vi "SetRange_XDM3051.vi"(7 "OFF_ON":T1, 8 "error in":errorcluster, 9 "AUTO":bool, 10 "Functions":T2, 11 "RS232_Input":refnum<visa-resource-name>) -> (0 "error out":errorcluster, 2 "response":string, 3 "RS232_Output":refnum<visa-resource-name>)   [LabVIEW 2017]
uses:
  controls/Functions_XDM3051.ctl
  controls/Off_On_XDM3051.ctl
panel:
  in  "Range":i32
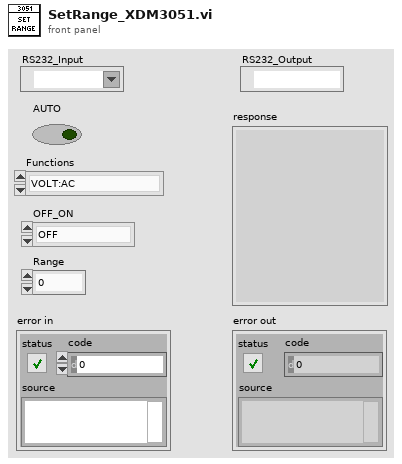
[diagram p1: front panel]
types:
  T1 = typedef "Off_On_XDM3051.ctl" = enum16{"OFF", "ON"}
  T2 = typedef "Functions_XDM3051.ctl" = enum16{"VOLT:AC", "VOLT:DC", "CURR:AC", "CURR:DC", "FREQ", "PER", "CAP", "CONT", "DIOD", "FRES", "RES", "TEMP:RTD"}
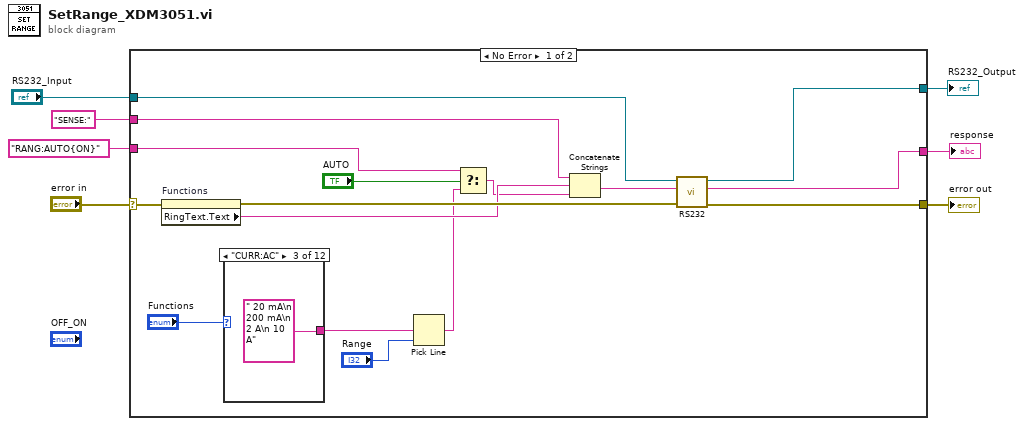
[diagram p0: block diagram]
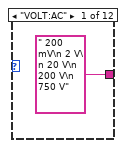
[diagram p2: hidden frame]
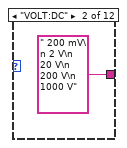
[diagram p3: hidden frame]
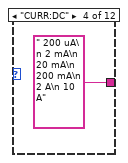
[diagram p4: hidden frame]
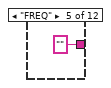
[diagram p5: hidden frame]
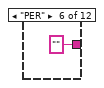
[diagram p6: hidden frame]
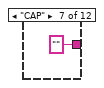
[diagram p7: hidden frame]
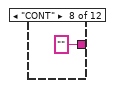
[diagram p8: hidden frame]
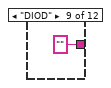
[diagram p9: hidden frame]
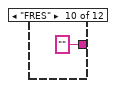
[diagram p10: hidden frame]
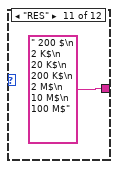
[diagram p11: hidden frame]
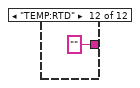
[diagram p12: hidden frame]
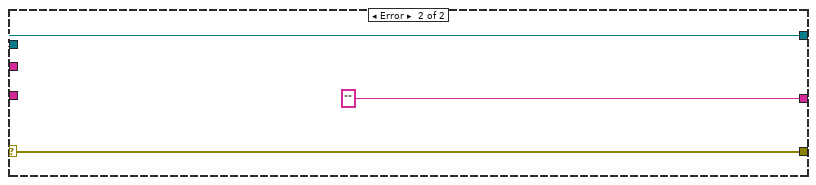
[diagram p13: hidden frame]
diagram:
  n1 = case shown="No Error" "error in" {
    selector: "error in" -> [w19 w38]
    tunnel: [w23 w38] -> w6
    tunnel: "RS232_Input" -> [w22 w37]
    tunnel: [w21 "" ("response")] -> w4
    tunnel: [w20 w37] -> w3
    tunnel: "SENSE:" ("command") -> [w12 _]
    tunnel: "RANG:AUTO{ON}" ("command") -> [w10 _]
    frame No Error {
      n2 = property on="Functions" class="Enum (strict)"(error in=w19) -> (error out=w18:errorcluster, "RingText.Text"=w11:string)  [unwired: 1 in, 1 out]
      n3 = case shown="\"CURR:AC\"" "Functions" {
        tunnel: [" 200 mV\n 2 V\n 20 V\n 200 V\n 750 V" " 200 mV\n 2 V\n 20 V\n 200 V\n 1000 V" " 20 mA\n 200 mA\n 2 A\n 10 A" " 200 uA\n 2 mA\n 20 mA\n 200 mA\n 2 A\n 10 A" "" "" "" "" "" "" " 200 $\n 2 K$\n 20 K$\n 200 K$\n 2 M$\n 10 M$\n 100 M$" ""] -> w13
        frame "VOLT:AC" {
        }
        frame "VOLT:DC" {
        }
        frame "CURR:AC" {
        }
        frame "CURR:DC" {
        }
        frame "FREQ" {
        }
        frame "PER" {
        }
        frame "CAP" {
        }
        frame "CONT" {
        }
        frame "DIOD" {
        }
        frame "FRES" {
        }
        frame "RES" {
        }
        frame "TEMP:RTD" {
        }
      }
      n4 = Pick Line(multi-line string=w13, line index="Range") -> (output string=w9:string)  [unwired: 1 in]
      n5 = Select(t=w10, s="AUTO", f=w9) -> (s? t:f=w8:string)
      n6 = Concatenate Strings(w12, w11, w8) -> (w17:string)
      n7 = call "RS232.vi"("error in"=w18, "command"=w17, "RS232_Input"=w22) -> ("error out"=w23:errorcluster, "response"=w21:string, "RS232_Output"=w20:refnum<visa-resource-name>)  [unwired: 6 in]
    }
    frame Error {
    }
  }
  "error out" <- w6
  "RS232_Output" <- w3
  "response" <- w4
